vi "LVITX OffsetMult Array.vi"(1 "XScale.Multiplier":dbl, 2 "XScale.Offset":dbl, 3 "Numeric":i32) -> (0 "Array":dbl[](array[numeric]))   [LabVIEW 2016, in "LVtoITX.lvclass"]
uses:
  LVtoITX.lvclass
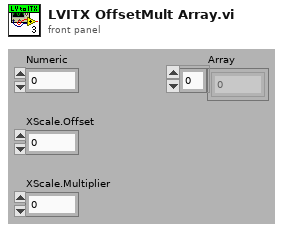
[diagram p1: front panel]
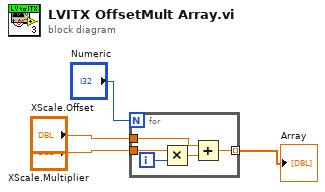
[diagram p0: block diagram]
diagram:
  n1 = for {
    N: "Numeric" -> [_]
    tunnel: "XScale.Multiplier" -> [w8]
    tunnel: "XScale.Offset" -> [w6]
    tunnel: [w5] -> w4 mode=indexing
    i -> [w9]
    n2 = Multiply(x=w8, y=w9) -> (x*y=w7:dbl)
    n3 = Add(x=w6, y=w7) -> (x+y=w5:dbl)
  }
  "Array" <- w4
